vi "playAudio.vi"(8 "error in":errorcluster) -> (0 "error out":errorcluster)   [LabVIEW 2020]
uses:
  clipOption.ctl
  <vilib>/measure/NI_MABase.lvlib
panel:
  in  "Enum":T1=enum."Scale Audio"
  in  "Source":enum32{"From WAV File", "Function Generator"}(tab)
  in  "WAV file path":path
  in  "Duplicate Left Channel?":bool
  in  "Samples per second":dbl
  in  "left signal type":T2(ring)
  in  "left frequency":dbl=10.0 format="%0.2p"
  in  "left amplitude":dbl=1.0 format="%0.2p"
  in  "left phase":dbl format="%.2p"
  in  "right signal type":T2(ring)
  in  "right frequency":dbl=10.0 format="%0.2p"
  in  "right amplitude":dbl=1.0 format="%0.2p"
  in  "right phase":dbl format="%.2p"
  in  "# seconds":dbl
  in  "Mono Audio?":bool
  in  "stop":bool
  in  "physical channels":tag="myDAQ1/audioOutputLeft, myDAQ1/audioOutputRight"
  # "Right Channel"
  # "Left Channel"
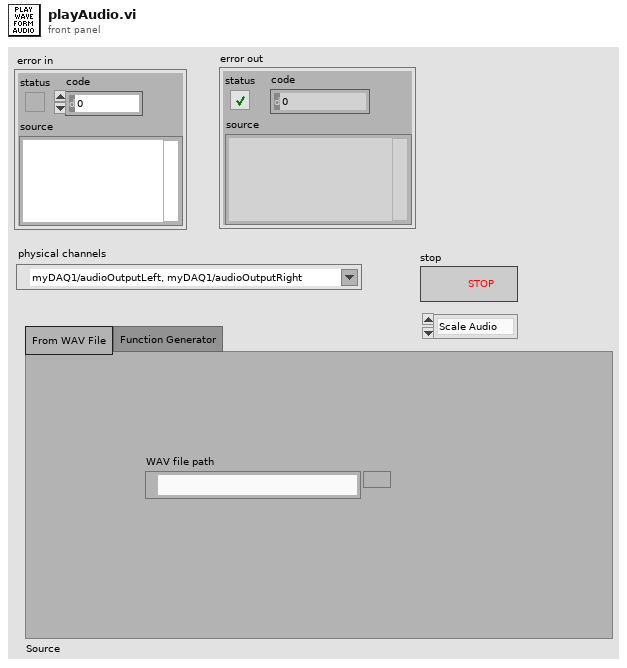
[diagram p1: front panel]
types:
  T1 = typedef "clipOption.ctl" = enum16{"Clip Audio", "Scale Audio"}
  T2 = enum16{"Sine Wave", "Triangle Wave", "Square Wave", "Sawtooth Wave"}
  T3 = enum8{"Enabled", "Disabled", "Disabled and Grayed Out"}
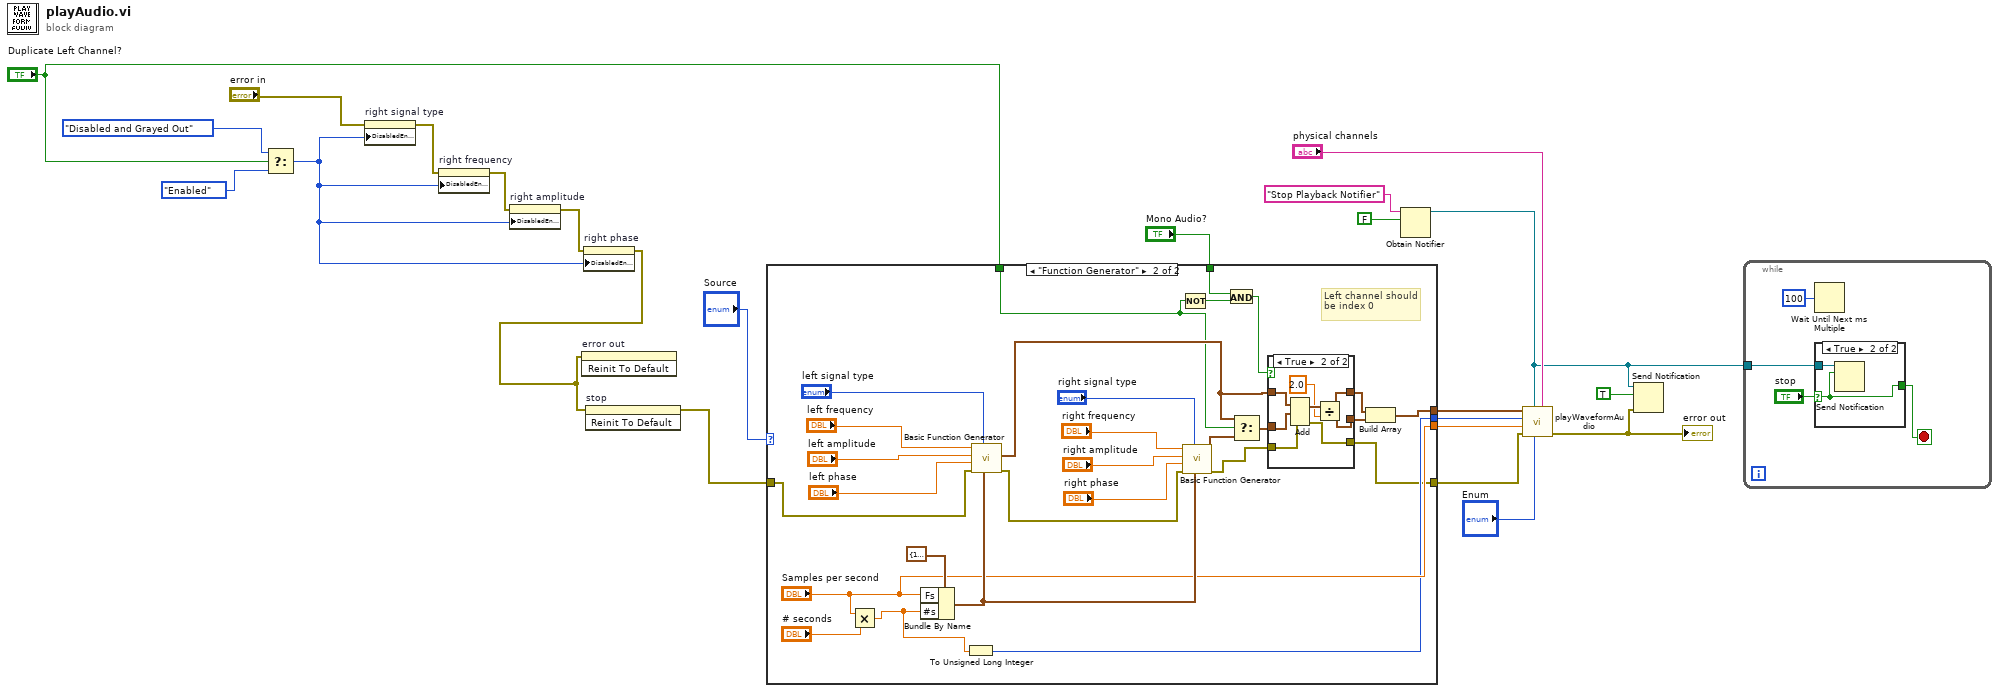
[diagram p0: block diagram]
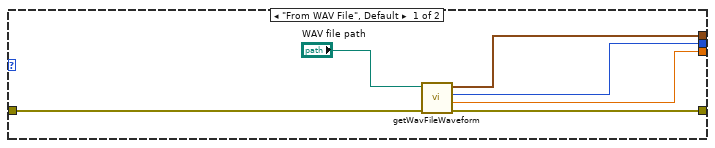
[diagram p2: hidden frame]
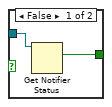
[diagram p4: hidden frame]
diagram:
  n1 = Select(t=T3."Disabled and Grayed Out" ("Disabled"), s="Duplicate Left Channel?", f=T3."Enabled" ("Disabled")) -> (s? t:f=w10:T3)
  n2 = property on="right signal type" class="Enum (strict)"(error in="error in", "DisabledEnum"=w10) -> (error out=w6:errorcluster)  [unwired: 1 in, 1 out]
  n3 = property on="right frequency" class="DigNum (strict)"(error in=w6, "DisabledEnum"=w10) -> (error out=w7:errorcluster)  [unwired: 1 in, 1 out]
  n4 = property on="right amplitude" class="DigNum (strict)"(error in=w7, "DisabledEnum"=w10) -> (error out=w8:errorcluster)  [unwired: 1 in, 1 out]
  n5 = property on="right phase" class="DigNum (strict)"(error in=w8, "DisabledEnum"=w10) -> (error out=w5:errorcluster)  [unwired: 1 in, 1 out]
  n6 = invoke on="error out" class="Clust (strict)" method="Reinit To Default"(error in=w5) -> ()  [unwired: 2 in, 3 out]
  n7 = invoke on="stop" class="Bool" method="Reinit To Default"(error in=w5) -> (error out=w16:errorcluster)  [unwired: 2 in, 2 out]
  n8 = case shown="\"Function Generator\"" "Source" {
    tunnel: [w28 w34] -> w23
    tunnel: [w27 "Samples per second"] -> w20
    tunnel: [w26 w47] -> w19
    tunnel: [w25 w40] -> w18
    tunnel: w16 -> [w24 w53]
    tunnel: "Duplicate Left Channel?" -> [_ w31]
    tunnel: "Mono Audio?" -> [_ w32]
    frame "From WAV File", Default {
      n9 = call "getWavFileWaveform.vi"("error in (no error)"=w24, "path to .WAV file"="WAV file path") -> ("error out"=w28:errorcluster, "sample rate (S/s)"=w27:dbl, "total number of samples/ch"=w25:u32, "audio waveform array"=w26:waveform(dbl)[])  [unwired: 4 in, 2 out]
    }
    frame "Function Generator" {
      # "Left channel should be index 0"
      n10 = Multiply(x="Samples per second", y="# seconds") -> (x*y=w41:dbl)
      n11 = Bundle By Name(cluster=cluster{"Fs":dbl, "#s":dbl} {"Fs"=1000.0, "#s"=1000.0} ("sampling"), "Fs"="Samples per second", "#s"=w41) -> (w44:cluster{"Fs":dbl, "#s":dbl})
      n12 = To Unsigned Long Integer(number=w41) -> (unsigned 32bit integer=w40:u32)
      n13 = call <vilib>:"Basic Function Generator.vi"("sampling info"=w44, "signal type"="left signal type", "error in (no error)"=w53, "phase"="left phase", "amplitude"="left amplitude", "frequency"="left frequency") -> ("error out"=w48:errorcluster, "signal out"=w39:waveform(dbl))  [unwired: 3 in, 1 out]
      n14 = Not(x=w31) -> (.not. x?=w33:bool)
      n15 = call <vilib>:"Basic Function Generator.vi"("sampling info"=w44, "signal type"="right signal type", "error in (no error)"=w48, "phase"="right phase", "amplitude"="right amplitude", "frequency"="right frequency") -> ("error out"=w35:errorcluster, "signal out"=w43:waveform(dbl))  [unwired: 3 in, 1 out]
      n16 = And(x=w32, y=w33) -> (x .and. y?=w30:bool)
      n17 = Select(t=w39, s=w31, f=w43) -> (s? t:f=w37:waveform(dbl))
      n18 = case shown="True" w30 {
        tunnel: w39 -> [w60 w67]
        tunnel: [w60 w61] -> w38
        tunnel: w37 -> [w59 w66]
        tunnel: [w59 w61] -> w36
        tunnel: w35 -> [w58 w65]
        tunnel: [w58 w64] -> w34
        frame False {
        }
        frame True {
          n19 = Add(1:w66, 2:w67, 4:w65) -> (0:w63:waveform(dbl), 3:w64:errorcluster)
          n20 = Divide(x=w63, y=2.0) -> (x/y=w61:waveform(dbl))
        }
      }
      n21 = Build Array(w38, w36) -> (w47:waveform(dbl)[])
    }
  }
  n22 = Obtain Notifier(name (unnamed)="Stop Playback Notifier", notification data type=FALSE) -> (notifier out=w4:refnum<notifier>)  [unwired: 2 in, 2 out]
  n23 = call "playWaveformAudio.vi"("physical channels"="physical channels", "Enum"="Enum", "stop playback notifier refnum"=w4, "error in (no error)"=w23, "sample rate (S/s)"=w20, "samples per channel"=w18, "input waveform array"=w19) -> ("error out"=w3:errorcluster)  [unwired: 4 in]
  "error out" <- w3
  n24 = Send Notification(notification=TRUE, notifier=w4, error in (no error)=w3) -> ()  [unwired: 2 out]
  n25 = while {
    tunnel: w4 -> [w70]
    stop <- w69 stop-if-true
    n26 = Wait Until Next ms Multiple(millisecond multiple=u32 100) -> ()  [unwired: 1 out]
    n27 = case shown="True" "stop" {
      selector: "stop" -> [_ w74]
      tunnel: w70 -> [w73 w75]
      tunnel: [w72 w74] -> w69
      frame False {
        n28 = Get Notifier Status(notifier=w73) -> (current notification=w72:bool)  [unwired: 1 in, 4 out]
      }
      frame True {
        n29 = Send Notification(notification=w74, notifier=w75) -> ()  [unwired: 1 in, 2 out]
      }
    }
  }
